vi "MCS_Jogging Control.vi"() -> ()   [LabVIEW 2010]
panel:
  out "Position (um)":dbl
  in  "?":bool
  in  "Jogging Step (um)":dbl
  in  "Channel":u32
  in  "Jog":bool
  in  "MCS System Locator":string
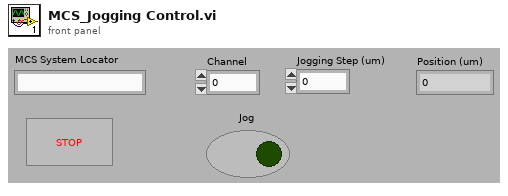
[diagram p1: front panel]
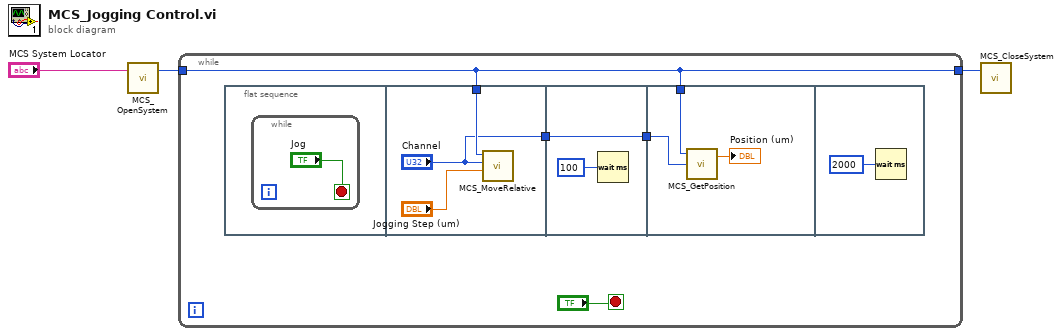
[diagram p0: block diagram]
diagram:
  n1 = call "MCS_OpenSystem.vi"("MCS System Locator"="MCS System Locator") -> ("System Index Out"=w2:u32)  [unwired: 1 in, 1 out]
  n2 = while {
    tunnel: [w6] -> w1
    tunnel: w2 -> [w6]
    stop <- "?" stop-if-true
    n3 = flat-sequence {
      tunnel: w6 -> [w11]
      tunnel: ["Channel"] -> w4
      tunnel: [w12] -> w5
      tunnel: w4 -> [w12]
      tunnel: w6 -> [w16]
      tunnel: w5 -> [w15]
      frame #0 {
        n4 = while {
          stop <- "Jog" stop-if-true
        }
      }
      frame #1 {
        n5 = call "MCS_MoveRelative.vi"("Moving Distance (um)"="Jogging Step (um)", "Channel Index In"="Channel", "System Index In"=w11) -> ()  [unwired: 1 in, 1 out]
      }
      frame #2 {
        n6 = Wait (ms)(milliseconds to wait=u32 100) -> ()  [unwired: 1 out]
      }
      frame #3 {
        n7 = call "MCS_GetPosition.vi"("Channel Index In"=w15, "System Index In"=w16) -> ("Position (um)"=→"Position (um)":dbl)  [unwired: 1 in, 1 out]
      }
      frame #4 {
        n8 = Wait (ms)(milliseconds to wait=u32 2000) -> ()  [unwired: 1 out]
      }
    }
  }
  n9 = call "MCS_CloseSystem.vi"("System Index In"=w1) -> ()  [unwired: 1 in, 1 out]
